vi "Day 12-Recursive Search.vi"(7 "Map":map{string, set{string}}(c390), 8 "Conditions":enum32{"Part 1", "Part 2"}(radio), 9 "Path in":string[](array[string]), 10 "Next Cave":string, 11 "Valid Paths in":set{string[]}(c389)) -> (3 "Valid Paths out":set{string[]}(c389))   [LabVIEW 2021]
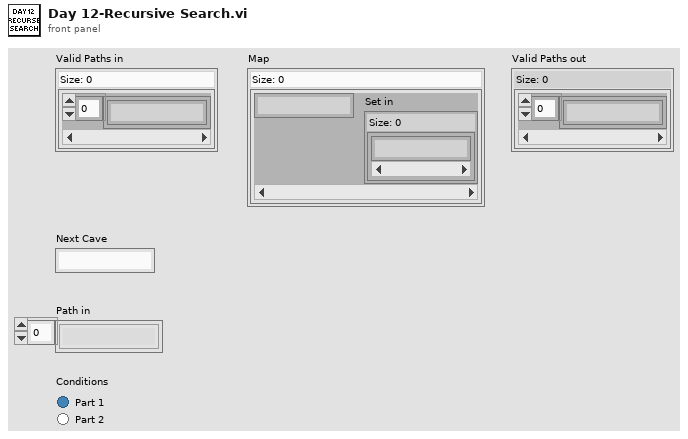
[diagram p1: front panel]
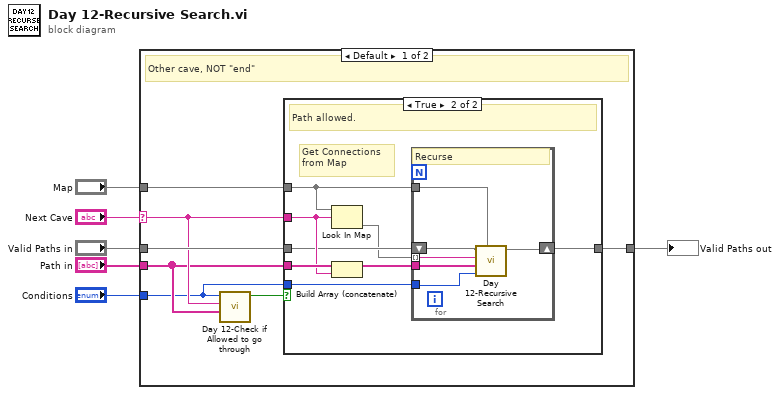
[diagram p0: block diagram]
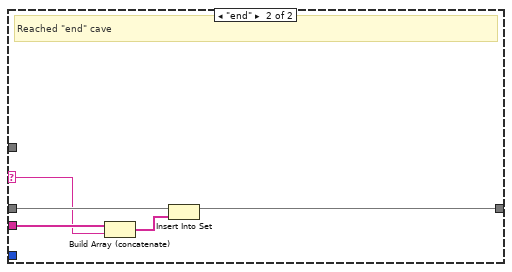
[diagram p3: hidden frame]
diagram:
  n1 = case shown="Default" "Next Cave" {
    selector: "Next Cave" -> [w9 w29]
    tunnel: "Map" -> [w10 _]
    tunnel: "Path in" -> [w8 w33]
    tunnel: "Valid Paths in" -> [w12 w32]
    tunnel: [w11 w30] -> w2
    tunnel: "Conditions" -> [w7 _]
    frame Default {
      # "Other cave, NOT \"end\""
      n2 = call "Day 12-Check if Allowed to go through.vi"("Path in"=w8, "Cave"=w9, "Conditions"=w7) -> ("Allowed?"=w13:bool)  [unwired: 8 in]
      n3 = case shown="True" w13 {
        tunnel: w10 -> [_ w22]
        tunnel: w9 -> [_ w19]
        tunnel: w8 -> [_ w21]
        tunnel: w12 -> [w14 w17]
        tunnel: [w14 w18] -> w11
        tunnel: w7 -> [_ w15]
        frame False {
          # "Path not allowed"
        }
        frame True {
          # "Get Connections from Map"
          # "Path allowed."
          n4 = Look In Map(map=w22, key=w19) -> (value=w16:set{string})  [unwired: 1 in, 1 out]
          n5 = Build Array (concatenate)(w21, w19) -> (w20:string[])
          n6 = for {
            tunnel: w22 -> [w27]
            tunnel: w16 -> [w28] mode=indexing
            tunnel: w20 -> [w24]
            shift-right: [w25] -> w18
            shift-left: w17 -> [w26]
            tunnel: w15 -> [w23]
            # "Recurse"
            n7 = call "Day 12-Recursive Search.vi"("Map"=w27, "Conditions"=w23, "Path in"=w24, "Next Cave"=w28, "Valid Paths in"=w26) -> ("Valid Paths out"=w25:set{string[]})  [unwired: 6 in]
          }
        }
      }
    }
    frame "end" {
      # "Reached \"end\" cave"
      n8 = Build Array (concatenate)(w33, w29) -> (w31:string[])
      n9 = Insert Into Set(10:w31, 11:w32) -> (3:w30:set{string[]})  [unwired: 1 out]
    }
  }
  "Valid Paths out" <- w2
